vi "Set TDMS File CPU and RAM Channel Properties.vi"(8 "error in (no error)":errorcluster, 10 "Logger Parameters":T1, 11 "Refnum in":refnum<k34>) -> (0 "error out":errorcluster, 3 "Refnum out":refnum<k34>)   [LabVIEW 2019, in "Telemetry Engine.lvlib"]
doc: "This VI sets the Physical Memory and CPU channel information along with their properties."
uses:
  Telemetry Engine.lvlib
  Types/Logger Data.ctl
  Types/System Channels.ctl
  Types/Target Info.ctl
  Shared/Constants.vi
  Shared/Telemetry Shared.lvlib
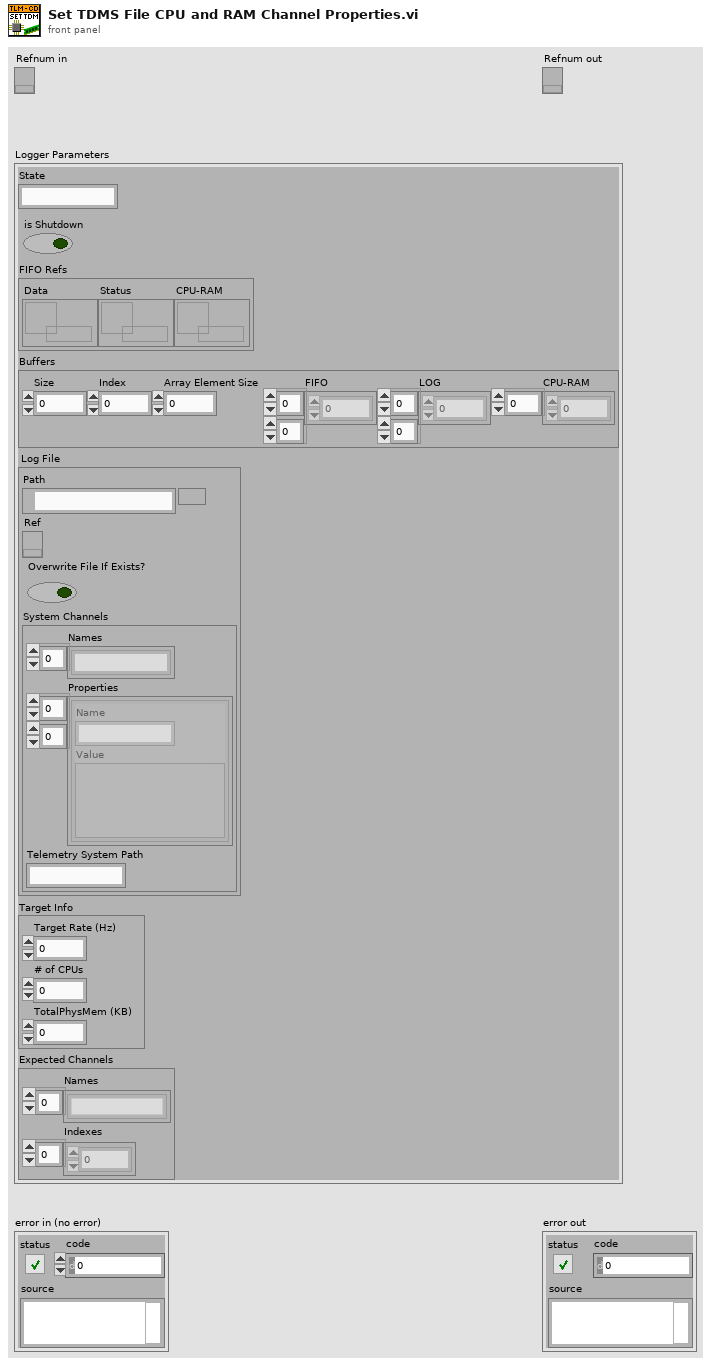
[diagram p1: front panel]
types:
  T1 = typedef "Telemetry Engine.lvlib/Logger Data.ctl" = cluster{"State":string, "is Shutdown":bool, "FIFO Refs":cluster{"Data":refnum<k33>, "Status":refnum<k33>, "CPU-RAM":refnum<k33>}, "Buffers":cluster{"Size":i32, "Index":i32, "Array Element Size":i32, "FIFO":dbl[][], "LOG":dbl[][], "CPU-RAM":dbl[]}, "Log File":cluster{"Path":path, "Ref":refnum<k34>, "Overwrite File If Exists?":bool, "System Channels":T2}, "Target Info":T3, "Expected Channels":cluster{"Names":string[], "Indexes":i32[]}}
  T2 = typedef "Telemetry Engine.lvlib/System Channels.ctl" = cluster{"Names":string[], "Properties":cluster{"Name":string, "Value":variant}[][], "Telemetry System Path":string}
  T3 = typedef "Telemetry Engine.lvlib/Target Info.ctl" = cluster{"Target Rate (Hz)":dbl, "# of CPUs":u32, "TotalPhysMem (KB)":dbl}
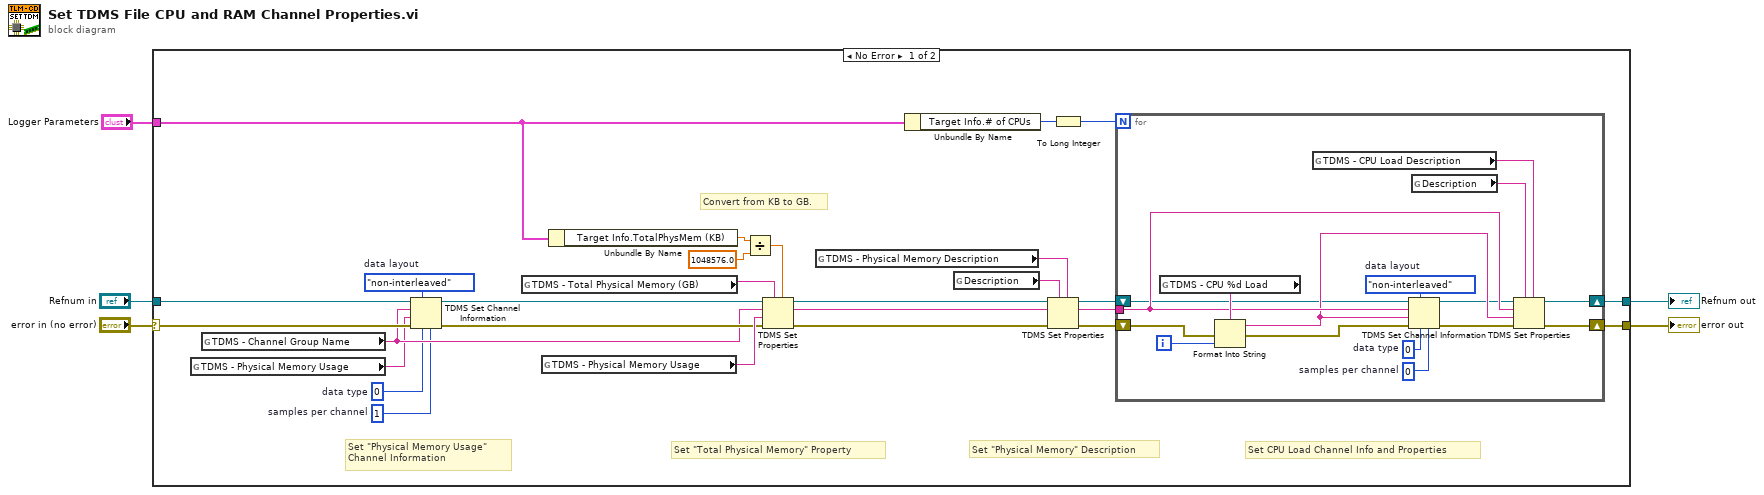
[diagram p0: block diagram]
diagram:
  n1 = case shown="No Error" "error in (no error)" {
    selector: "error in (no error)" -> [w23 w50]
    tunnel: "Logger Parameters" -> [w11 _]
    tunnel: "Refnum in" -> [w21 w49]
    tunnel: [w6 w49] -> w4
    tunnel: [w12 w50] -> w3
    frame No Error {
      w16 = u32 1  # samples per channel
      w17 = i8 0  # data type
      w19 = enum16{"non-interleaved", "interleaved"}."non-interleaved"  # data layout
      # "Set CPU Load Channel Info and Properties"
      # "Set \"Physical Memory\" Description"
      # "Set \"Physical Memory Usage\" Channel Information"
      # "Set \"Total Physical Memory\" Property"
      # "Convert from KB to GB."
      n2 = global read "Constants.vi" "TDMS - Physical Memory Usage"() -> (w18:string)
      n3 = global read "Constants.vi" "TDMS - Channel Group Name"() -> (w20:string)
      n4 = TDMS Set Channel Information(4:w16, 6:w17, 7:w19, 8:w23, 9:w18, 10:w20, 11:w21) -> (0:w24:errorcluster, 3:w22:refnum<k34>)
      n5 = global read "Constants.vi" "TDMS - Total Physical Memory (GB)"() -> (w32:string)
      n6 = global read "Constants.vi" "TDMS - Physical Memory Usage"() -> (w28:string)
      n7 = Unbundle By Name(w11) -> ("Target Info.TotalPhysMem (KB)"=w27:dbl)
      n8 = Divide(x=w27, y=1048576.0) -> (x/y=w25:dbl)
      n9 = TDMS Set Properties(5:w25, 7:w32, 8:w24, 9:w28, 10:w20, 11:w22) -> (0:w30:errorcluster, 2:w29:string, 3:w31:refnum<k34>)  [unwired: 1 out]
      n10 = global read "Constants.vi" "TDMS - Physical Memory Description"() -> (w14:string)
      n11 = Unbundle By Name(w11) -> ("Target Info.# of CPUs"=w10:u32)
      n12 = global read "Constants.vi" "Description"() -> (w15:string)
      n13 = TDMS Set Properties(5:w14, 7:w15, 8:w30, 10:w29, 11:w31) -> (0:w13:errorcluster, 2:w8:string, 3:w7:refnum<k34>)  [unwired: 1 in, 1 out]
      n14 = To Long Integer(number=w10) -> (32bit integer=w9:i32)
      n15 = for {
        N: w9 -> [_]
        shift-right: [w47] -> w12
        shift-left: w13 -> [w42]
        tunnel: w8 -> [w39]
        shift-right: [w35] -> w6
        shift-left: w7 -> [w37]
        i -> [w40]
        w44 = enum16{"non-interleaved", "interleaved"}."non-interleaved"  # data layout
        w45 = u8 0  # data type
        w46 = u32 0  # samples per channel
        n16 = global read "Constants.vi" "TDMS - CPU %d Load"() -> (w43:string)
        n17 = Format Into String(format string=w43, error in=w42, w40) -> (resulting string=w38:string, error out=w41:errorcluster)  [unwired: 1 in]
        n18 = global read "Constants.vi" "TDMS - CPU Load Description"() -> (w33:string)
        n19 = TDMS Set Channel Information(4:w46, 6:w45, 7:w44, 8:w41, 9:w38, 10:w39, 11:w37) -> (0:w48:errorcluster, 3:w36:refnum<k34>)
        n20 = global read "Constants.vi" "Description"() -> (w34:string)
        n21 = TDMS Set Properties(5:w33, 7:w34, 8:w48, 9:w38, 10:w39, 11:w36) -> (0:w47:errorcluster, 3:w35:refnum<k34>)  [unwired: 2 out]
      }
    }
    frame Error {
    }
  }
  "Refnum out" <- w4
  "error out" <- w3
